vi "test-cubic-spline-00.vi"() -> ()   [LabVIEW 2019]
uses:
  <vilib>/Rock Robotics/WPI/ThirdParty/JAS_Junk/TrajLib/POSEwCURVATURE.ctl
  <vilib>/Rock Robotics/WPI/ThirdParty/JAS_Junk/TrajLib/POSE2D.ctl
  <vilib>/Rock Robotics/WPI/ThirdParty/JAS_Junk/TrajLib/TRANSLATION2D.ctl
  <vilib>/Rock Robotics/WPI/ThirdParty/JAS_Junk/TrajLib/ROTATION2D.ctl
  <vilib>/Rock Robotics/WPI/ThirdParty/JAS_Junk/TrajLib/Rotation_CreateAngle.vi
  <vilib>/Rock Robotics/WPI/ThirdParty/JAS_Junk/TrajLib/Util_CalcDist.vi
  <vilib>/Rock Robotics/WPI/ThirdParty/JAS_Junk/TrajLib/Trajectory_Library.lvlib
panel:
  out "XY Graph":cluster{dbl[], dbl[]}(graph)
  out "All Interior \nwayPoints\nFound (True)":bool
  out "end rot = 0":dbl
  out "end y = 0":dbl
  out "end x = 0":dbl
  out "start rot = 0":dbl
  out "start y = 0":dbl
  out "start x = 0":dbl
  out "max dtheta < 0.0872":dbl
  out "max dy < 0.00127":dbl
  out "max dx  < 0.127":dbl
  out "Overall Error":errorcluster
  out "Elements":i32
  out "Create Spline Error":errorcluster
  out "SplinePoses\nWCurve":T1[](array[typedef]) {"POSE"."ROTATION"."SIN" format="%13.4f"; "POSE"."ROTATION"."COS" format="%13.4f"; "POSE"."ROTATION"."VALUE" format="%13.4f"; "POSE"."TRANSLATION"."Y" format="%14.3f"; "POSE"."TRANSLATION"."X" format="%14.3f"}
  out "Elapsed Time":dbl
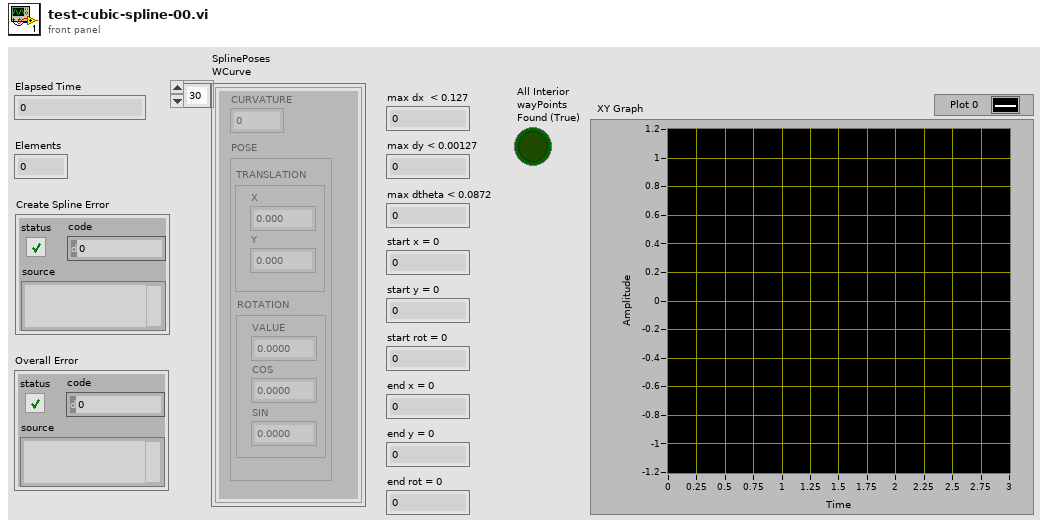
[diagram p1: front panel]
types:
  T1 = typedef "Trajectory_Library.lvlib/POSEwCURVATURE.ctl" = cluster{"CURVATURE":dbl, "POSE":T2}
  T2 = typedef "Trajectory_Library.lvlib/POSE2D.ctl" = cluster{"TRANSLATION":T3, "ROTATION":T4}
  T3 = typedef "Trajectory_Library.lvlib/TRANSLATION2D.ctl" = cluster{"X":dbl, "Y":dbl}
  T4 = typedef "Trajectory_Library.lvlib/ROTATION2D.ctl" = cluster{"VALUE":dbl, "COS":dbl, "SIN":dbl}
  T5 = typedef "Trajectory_Library.lvlib/SPLINE_CTRL_VECTOR.ctl" = cluster{"Xs":dbl[], "Ys":dbl[]}
  T6 = typedef "Trajectory_Library.lvlib/SPLINE.ctl" = cluster{"Degree":i32, "Coefficients":T7}
  T7 = typedef "NI_Matrix.lvlib/RealMatrix.ctl" = dbl[][]
  T8 = typedef "Trajectory_Library.lvlib/TWIST2D.ctl" = cluster{"dX":dbl, "dY":dbl, "dTHETA":dbl}
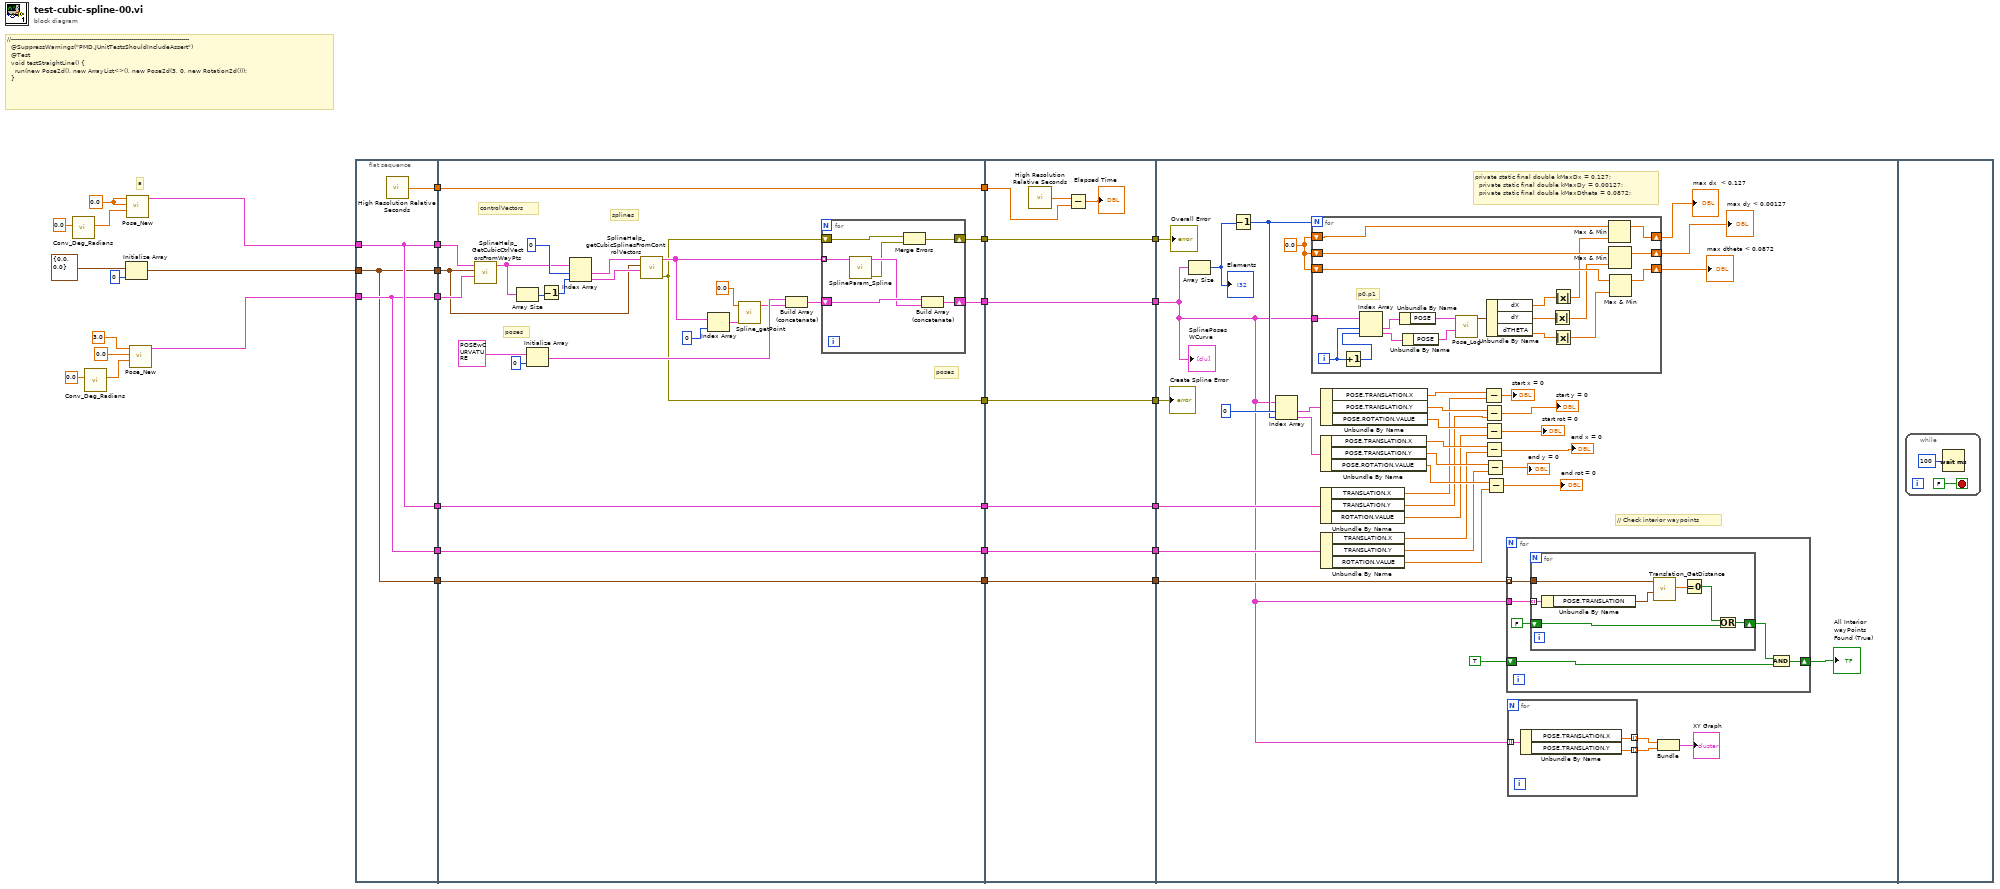
[diagram p0: block diagram]
diagram:
  w8 = 0.0 ("X")
  # "a"
  # "//-----------------------------------------------------------------------------------------\n  @SuppressWarnings(\"PMD.JUnitTestsShouldIncludeAssert\")\n  @Test\n  void testStraightLine() {\n    run(new Pose2d(), new ArrayList<>(), new Pose2d(3, 0, new Rotation2d()));\n  }"
  n1 = call <vilib>:"Conv_Deg_Radians.vi"("Degress"=0.0) -> ("Radians"=w7:dbl)  [unwired: 10 in]
  n2 = call <vilib>:"Conv_Deg_Radians.vi"("Degress"=0.0) -> ("Radians"=w4:dbl)  [unwired: 10 in]
  n3 = Initialize Array(T3 {"X"=0.0, "Y"=0.0} ("TRANSLATION"), 0 ("dimension size")) -> (w1:T3[])
  n4 = call <vilib>:"Pose_New.vi"("Heading"=w7, "Y"=w8, "X"=w8) -> ("out POSe"=w30:T2)  [unwired: 8 in]
  n5 = call <vilib>:"Pose_New.vi"("Heading"=w4, "Y"=0.0, "X"=3.0) -> ("out POSe"=w27:T2)  [unwired: 8 in]
  n6 = flat-sequence {
    tunnel: w30 -> [w35]
    tunnel: [w35] -> w29
    tunnel: w1 -> [w33]
    tunnel: [w33] -> w28
    tunnel: w27 -> [w34]
    tunnel: [w34] -> w26
    tunnel: [w36] -> w25
    tunnel: [w35] -> w17
    tunnel: [w34] -> w14
    tunnel: [w33] -> w9
    tunnel: w29 -> [w61]
    tunnel: w28 -> [w53]
    tunnel: w26 -> [w60]
    tunnel: [w52] -> w24
    tunnel: w25 -> [w52]
    tunnel: [w42] -> w23
    tunnel: [w41] -> w21
    tunnel: [w40] -> w19
    tunnel: w17 -> [w39]
    tunnel: [w39] -> w16
    tunnel: w14 -> [w38]
    tunnel: [w38] -> w13
    tunnel: [w37] -> w10
    tunnel: w9 -> [w37]
    tunnel: w24 -> [w77]
    tunnel: w23 -> [w76]
    tunnel: [w76] -> w22
    tunnel: w21 -> [w75]
    tunnel: [w75] -> w20
    tunnel: w19 -> [w74]
    tunnel: [w74] -> w18
    tunnel: w16 -> [w71]
    tunnel: [w71] -> w15
    tunnel: w13 -> [w70]
    tunnel: [w70] -> w12
    tunnel: [w69] -> w11
    tunnel: w10 -> [w69]
    tunnel: w22 -> [w78]
    tunnel: w20 -> [w115]
    tunnel: w18 -> [w114]
    tunnel: w15 -> [w108]
    tunnel: w12 -> [w107]
    tunnel: w11 -> [w84]
    frame #0 {
      n7 = call <vilib>:"High Resolution Relative Seconds.vi"() -> ("relative seconds"=w36:dbl)
    }
    frame #1 {
      # "poses"
      # "poses"
      # "splines"
      # "controlVectors"
      n8 = call <vilib>:"SplineHelp_GetCubicCtrlVectorsFromWayPts.vi"("Enging POSE"=w60, "Interior WAYPOINTS"=w53, "Starting POSE"=w61) -> ("SplineControlVectors"=w57:T5[])  [unwired: 8 in]
      n9 = Array Size(array=w57) -> (size(s)=w58:i32)
      n10 = Initialize Array(T1 {"CURVATURE"=0.0, "POSE"={"TRANSLATION"={"X"=0.0, "Y"=0.0}, "ROTATION"={"VALUE"=0.0, "COS"=1.0, "SIN"=0.0}}} ("POSEwCURVATURE"), 0 ("dimension size")) -> (w46:T1[])
      n11 = Decrement(x=w58) -> (x-1=w56:i32)
      n12 = Index Array(array=w57, index #1=0 ("index"), index #2=w56) -> (element #1=w55:T5, element #2=w54:T5)
      n13 = call <vilib>:"SplineHelp_getCubicSplinesFromControlVectors.vi"("endCtrlVector"=w54, "InternalWaypoints"=w53, "startCtrlVector"=w55) -> ("error out"=w41:errorcluster, "splines"=w43:T6[])  [unwired: 3 in, 4 out]
      n14 = Index Array(array=w43, index=0) -> (element=w48:T6)
      n15 = call <vilib>:"Spline_getPoint.vi"("inputSPLINE"=w48, "Time"=0.0) -> ("POSEwCURVATURE"=w45:T1)  [unwired: 9 in]
      n16 = Build Array (concatenate)(w46, w45) -> (w44:T1[])
      n17 = for {
        shift-right: [w65] -> w42
        shift-left: w44 -> [w67]
        tunnel: w43 -> [w68] mode=indexing
        shift-right: [w63] -> w40
        shift-left: w41 -> [w64]
        n18 = call <vilib>:"SplineParam_Spline.vi"("inputSPLINE"=w68) -> ("error out"=w62:errorcluster, "outputPOSEwCURVATURE"=w66:T1[])  [unwired: 9 in]
        n19 = Merge Errors(w64, w62) -> (w63:errorcluster)
        n20 = Build Array (concatenate)(w67, w66) -> (w65:T1[])
      }
    }
    frame #2 {
      n21 = call <vilib>:"High Resolution Relative Seconds.vi"() -> ("relative seconds"=w72:dbl)
      n22 = Subtract(x=w72, y=w77) -> (x-y=→"Elapsed Time":dbl)
    }
    frame #3 {
      w112 = 0.0
      # "// Check interior waypoints"
      # "private static final double kMaxDx = 0.127;\n  private static final double kMaxDy = 0.00127;\n  private static final double kMaxDtheta = 0.0872;"
      n23 = Array Size(array=w78) -> (size(s)=w113:i32)
      "Elements" <- w113
      n24 = Decrement(x=w113) -> (x-1=w105:i32)
      n25 = Index Array(array=w78, index #1=0 ("index"), index #2=w105) -> (element #1=w104:T1, element #2=w103:T1)
      n26 = for {
        N: w105 -> [_]
        tunnel: w78 -> [w149]
        shift-right: [w140] -> w111
        shift-left: w112 -> [w137]
        shift-right: [w138] -> w109
        shift-left: w112 -> [w135]
        shift-right: [w139] -> w110
        shift-left: w112 -> [w136]
        i -> [w151]
        # "p0,p1"
        n27 = Increment(x=w151) -> (x+1=w150:i32)
        n28 = Index Array(array=w149, index #1=w151, index #2=w150) -> (element #1=w148:T1, element #2=w147:T1)
        n29 = Unbundle By Name(w148) -> ("POSE"=w146:T2)
        n30 = Unbundle By Name(w147) -> ("POSE"=w145:T2)
        n31 = call <vilib>:"Pose_Log.vi"("end POSE"=w145, "in POSE"=w146) -> ("out TWIST"=w144:T8)  [unwired: 9 in]
        n32 = Unbundle By Name(w144) -> ("dX"=w141:dbl, "dY"=w142:dbl, "dTHETA"=w143:dbl)
        n33 = Absolute Value(x=w142) -> (abs(x)=w133:dbl)
        n34 = Absolute Value(x=w141) -> (abs(x)=w134:dbl)
        n35 = Absolute Value(x=w143) -> (abs(x)=w132:dbl)
        n36 = Max & Min(x=w137, y=w134) -> (max(x,y)=w140:dbl)  [unwired: 1 out]
        n37 = Max & Min(x=w136, y=w133) -> (max(x,y)=w139:dbl)  [unwired: 1 out]
        n38 = Max & Min(x=w135, y=w132) -> (max(x,y)=w138:dbl)  [unwired: 1 out]
      }
      "max dx  < 0.127" <- w111
      "max dy < 0.00127" <- w110
      "max dtheta < 0.0872" <- w109
      n39 = Unbundle By Name(w103) -> ("POSE.TRANSLATION.X"=w99:dbl, "POSE.TRANSLATION.Y"=w98:dbl, "POSE.ROTATION.VALUE"=w97:dbl)
      n40 = Unbundle By Name(w108) -> ("TRANSLATION.X"=w96:dbl, "TRANSLATION.Y"=w95:dbl, "ROTATION.VALUE"=w94:dbl)
      n41 = Unbundle By Name(w104) -> ("POSE.TRANSLATION.X"=w102:dbl, "POSE.TRANSLATION.Y"=w101:dbl, "POSE.ROTATION.VALUE"=w100:dbl)
      n42 = Unbundle By Name(w107) -> ("TRANSLATION.X"=w93:dbl, "TRANSLATION.Y"=w92:dbl, "ROTATION.VALUE"=w91:dbl)
      n43 = Subtract(x=w102, y=w96) -> (x-y=→"start x = 0":dbl)
      n44 = Subtract(x=w101, y=w95) -> (x-y=→"start y = 0":dbl)
      n45 = Subtract(x=w100, y=w94) -> (x-y=→"start rot = 0":dbl)
      n46 = Subtract(x=w99, y=w93) -> (x-y=→"end x = 0":dbl)
      n47 = Subtract(x=w98, y=w92) -> (x-y=→"end y = 0":dbl)
      n48 = Subtract(x=w97, y=w91) -> (x-y=→"end rot = 0":dbl)
      n49 = for {
        tunnel: w84 -> [w119] mode=indexing
        tunnel: w78 -> [w124]
        shift-right: [w123] -> w82
        shift-left: TRUE -> [w122]
        n50 = for {
          tunnel: w124 -> [w128] mode=indexing
          shift-right: [w131] -> w120
          shift-left: FALSE -> [w130]
          tunnel: w119 -> [w129]
          n51 = Unbundle By Name(w128) -> ("POSE.TRANSLATION"=w127:T3)
          n52 = call <vilib>:"Translation_GetDistance.vi"("other Translation"=w127, "In Translation"=w129) -> ("Distance"=w126:dbl)  [unwired: 9 in]
          n53 = Equal To 0?(x=w126) -> (x = 0?=w125:bool)
          n54 = Or(x=w125, y=w130) -> (x .or. y?=w131:bool)
        }
        n55 = And(x=w120, y=w122) -> (x .and. y?=w123:bool)
      }
      "All Interior \nwayPoints\nFound (True)" <- w82
      n56 = for {
        tunnel: [w118] -> w81 mode=indexing
        tunnel: [w117] -> w80 mode=indexing
        tunnel: w78 -> [w116] mode=indexing
        n57 = Unbundle By Name(w116) -> ("POSE.TRANSLATION.X"=w118:dbl, "POSE.TRANSLATION.Y"=w117:dbl)
      }
      n58 = Bundle(w81, w80) -> (→"XY Graph":cluster{dbl[], dbl[]})  [unwired: 1 in]
      "SplinePoses\nWCurve" <- w78
      "Create Spline Error" <- w115
      "Overall Error" <- w114
    }
    frame #4 {
      n59 = while {
        stop <- FALSE stop-if-true
        n60 = Wait (ms)(milliseconds to wait=u32 100) -> ()  [unwired: 1 out]
      }
    }
  }
